vi "Valid Crossings.vi"(8 "Input Valid?":bool, 9 "Value In":fxp<+,32,16> format="%#_21g", 11 "Reference":fxp<+,32,16> format="%#_21g") -> (3 "Value Out":fxp<+,32,16> format="%#_21g")   [LabVIEW 2013]
uses:
  <vilib>/rvi/FXPMathLib/FxpMul/XNode/nifxpmath_Multiplier.xnode
  <vilib>/rvi/FXPMathLib/sim/FxpSim.dll
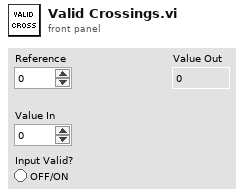
[diagram p1: front panel]
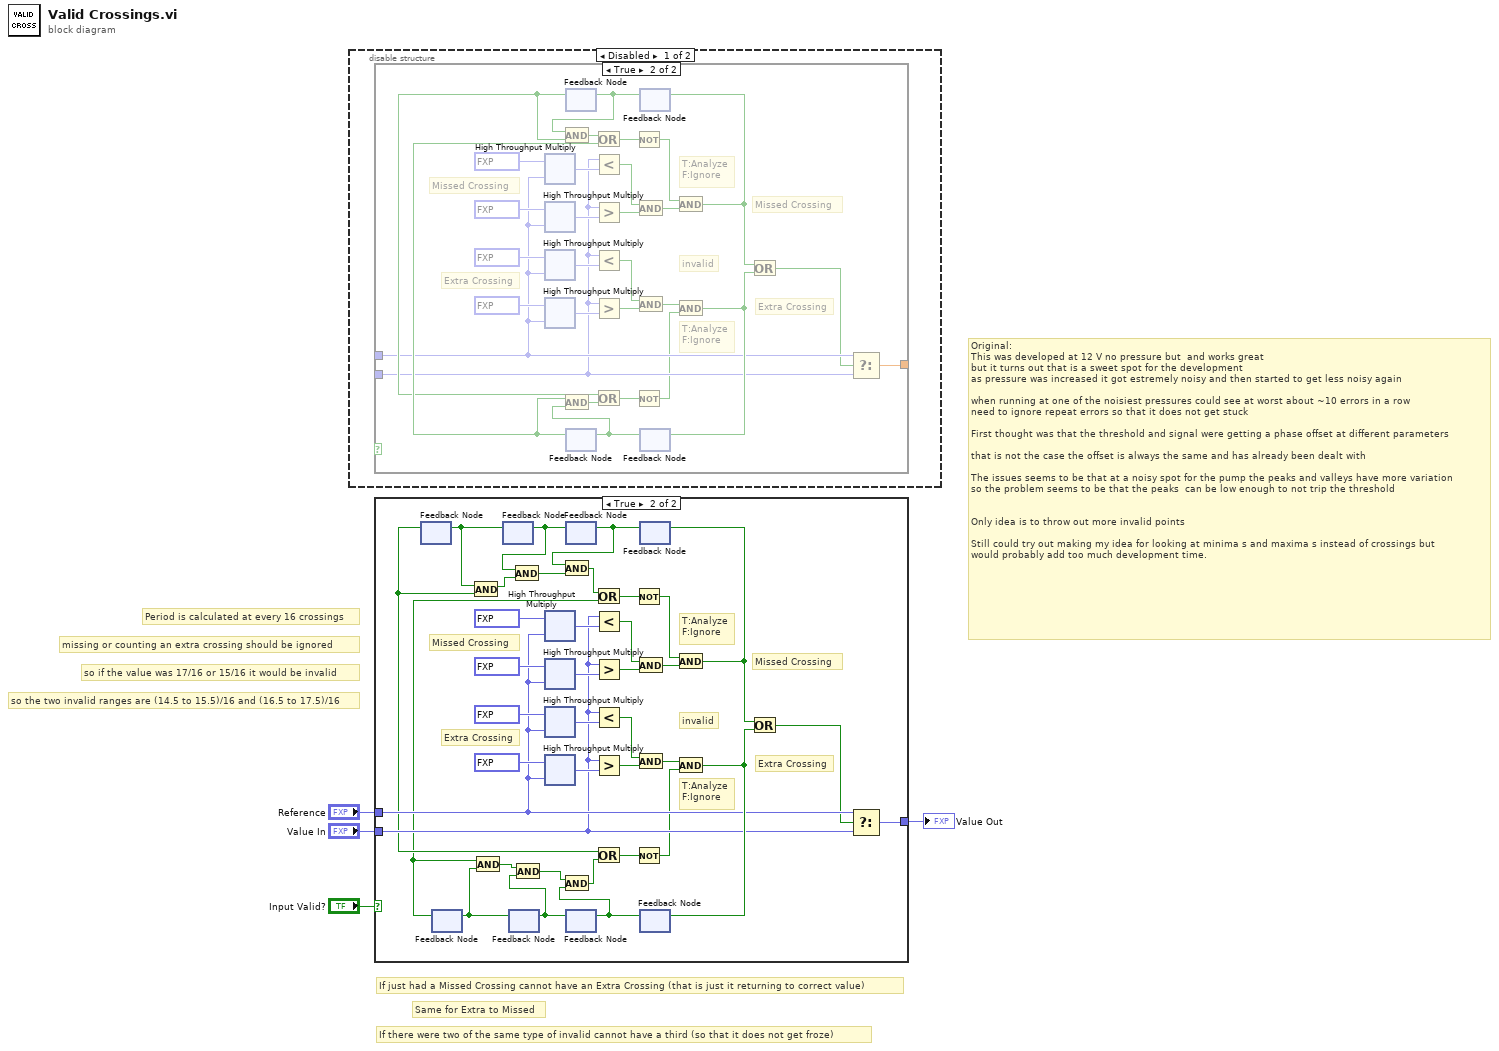
[diagram p0: block diagram]
diagram:
  # "Original:\nThis was developed at 12 V no pressure but  and works great\nbut it turns out that is a sweet spot for the development\nas pressure was increased it got estremely noisy and then started to get less noisy again\n\nwhen running at one of the noisiest pressures could see at worst about ~10 errors in a row\nneed to ignore repeat errors so that it does not get stuck\n\nFirst thought was that the threshold and signal were getting a phase offset at different parameters\n\nthat is not the case the offset is always the same and has already been dealt with\n\nThe issues seems to be that at a noisy spot for the pump the peaks and valleys have more variation\nso the problem seems to be that the peaks  can be low enough to not trip the threshold\n\n\nOnly idea is to throw out more invalid points\n\nStill could try out making my idea for looking at minima s and maxima s instead of crossings but\nwould probably add too much development time."
  # "If there were two of the same type of invalid cannot have a third (so that it does not get froze)"
  # "Same for Extra to Missed"
  # "If just had a Missed Crossing cannot have an Extra Crossing (that is just it returning to correct value)"
  # "so the two invalid ranges are (14.5 to 15.5)/16 and (16.5 to 17.5)/16"
  # "so if the value was 17/16 or 15/16 it would be invalid"
  # "missing or counting an extra crossing should be ignored"
  # "Period is calculated at every 16 crossings"
  n1 = disable-structure shown="Disabled" {
    frame Disabled {
      n2 = case shown="True" {
        selector: _ -> [_ _]
        tunnel: _ -> [w5 w13]
        tunnel: _ -> [_ w11]
        tunnel: [w5 w10] -> _
        frame False {
        }
        frame True {
          # "Missed Crossing"
          # "Extra Crossing"
          # "T:Analyze\nF:Ignore"
          # "T:Analyze\nF:Ignore"
          # "Extra Crossing"
          # "Missed Crossing"
          # "invalid"
          n3 = xnode ("High Throughput Multiply")("x"=fxp<+,6,1> 1.09375, "y"=w13) -> ("x*y"=w31:fxp<+,38,17>)
          n4 = xnode ("High Throughput Multiply")("x"=fxp<+,6,1> 1.03125, "y"=w13) -> ("x*y"=w30:fxp<+,38,17>)
          n5 = xnode ("High Throughput Multiply")("x"=fxp<+,6,1> 0.96875, "y"=w13) -> ("x*y"=w29:fxp<+,38,17>)
          n6 = xnode ("High Throughput Multiply")("x"=fxp<+,6,1> 0.90625, "y"=w13) -> ("x*y"=w28:fxp<+,38,17>)
          n7 = feedback #1() -> (w14:bool)  [unwired: 1 in]
          n8 = feedback #2() -> (w17:bool)  [unwired: 1 in]
          n9 = Less?(x=w11, y=w31) -> (x < y?=w26:bool)
          n10 = Greater?(x=w11, y=w30) -> (0:w27:bool)
          n11 = Less?(x=w11, y=w29) -> (x < y?=w25:bool)
          n12 = Greater?(x=w11, y=w28) -> (0:w24:bool)
          n13 = And(x=w26, y=w27) -> (x .and. y?=w22:bool)
          n14 = And(x=w25, y=w24) -> (x .and. y?=w23:bool)
          n15 = feedback #3() -> (w15:bool)  [unwired: 1 in]
          n16 = And(x=w15, y=w14) -> (x .and. y?=w19:bool)
          n17 = feedback-in #1(w15) -> ()
          n18 = Or(x=w19, y=w17) -> (x .or. y?=w9:bool)
          n19 = Not(x=w9) -> (.not. x?=w6:bool)
          n20 = feedback #4() -> (w16:bool)  [unwired: 1 in]
          n21 = And(x=w17, y=w16) -> (x .and. y?=w18:bool)
          n22 = feedback-in #2(w16) -> ()
          n23 = Or(x=w14, y=w18) -> (x .or. y?=w8:bool)
          n24 = Not(x=w8) -> (.not. x?=w7:bool)
          n25 = And(x=w6, y=w22) -> (x .and. y?=w20:bool)
          n26 = feedback-in #3(w20) -> ()
          n27 = And(x=w23, y=w7) -> (x .and. y?=w21:bool)
          n28 = feedback-in #4(w21) -> ()
          n29 = Or(x=w20, y=w21) -> (x .or. y?=w12:bool)
          n30 = Select(t=w13, s=w12, f=w11) -> (s? t:f=w10:dbl)
        }
      }
    }
    frame Enabled {
    }
  }
  n31 = case shown="True" "Input Valid?" {
    tunnel: "Reference" -> [w36 w54]
    tunnel: "Value In" -> [_ w52]
    tunnel: [w36 w51] -> w2
    frame False {
    }
    frame True {
      # "Missed Crossing"
      # "Extra Crossing"
      # "T:Analyze\nF:Ignore"
      # "T:Analyze\nF:Ignore"
      # "Extra Crossing"
      # "Missed Crossing"
      # "invalid"
      n32 = feedback #5() -> (w46:bool)  [unwired: 1 in]
      n33 = feedback #6() -> (w41:bool)  [unwired: 1 in]
      n34 = feedback #7() -> (w45:bool)  [unwired: 1 in]
      n35 = feedback-in #5(w45) -> ()
      n36 = And(x=w45, y=w46) -> (x .and. y?=w43:bool)
      n37 = feedback #8() -> (w40:bool)  [unwired: 1 in]
      n38 = feedback-in #6(w40) -> ()
      n39 = And(x=w41, y=w40) -> (x .and. y?=w38:bool)
      n40 = xnode ("High Throughput Multiply")("x"=fxp<+,6,1> 1.09375, "y"=w54) -> ("x*y"=w70:fxp<+,38,17>)
      n41 = xnode ("High Throughput Multiply")("x"=fxp<+,6,1> 1.03125, "y"=w54) -> ("x*y"=w69:fxp<+,38,17>)
      n42 = xnode ("High Throughput Multiply")("x"=fxp<+,6,1> 0.96875, "y"=w54) -> ("x*y"=w68:fxp<+,38,17>)
      n43 = xnode ("High Throughput Multiply")("x"=fxp<+,6,1> 0.90625, "y"=w54) -> ("x*y"=w67:fxp<+,38,17>)
      n44 = feedback #9() -> (w44:bool)  [unwired: 1 in]
      n45 = feedback-in #7(w44) -> ()
      n46 = And(x=w44, y=w43) -> (x .and. y?=w42:bool)
      n47 = feedback #10() -> (w39:bool)  [unwired: 1 in]
      n48 = feedback-in #8(w39) -> ()
      n49 = And(x=w38, y=w39) -> (x .and. y?=w37:bool)
      n50 = Less?(x=w52, y=w70) -> (x < y?=w65:bool)
      n51 = Greater?(x=w52, y=w69) -> (0:w66:bool)
      n52 = Less?(x=w52, y=w68) -> (x < y?=w64:bool)
      n53 = Greater?(x=w52, y=w67) -> (0:w63:bool)
      n54 = And(x=w65, y=w66) -> (x .and. y?=w61:bool)
      n55 = And(x=w64, y=w63) -> (x .and. y?=w62:bool)
      n56 = feedback #11() -> (w55:bool)  [unwired: 1 in]
      n57 = And(x=w55, y=w42) -> (x .and. y?=w58:bool)
      n58 = feedback-in #9(w55) -> ()
      n59 = Or(x=w58, y=w41) -> (x .or. y?=w50:bool)
      n60 = Not(x=w50) -> (.not. x?=w47:bool)
      n61 = feedback #12() -> (w56:bool)  [unwired: 1 in]
      n62 = And(x=w37, y=w56) -> (x .and. y?=w57:bool)
      n63 = feedback-in #10(w56) -> ()
      n64 = Or(x=w46, y=w57) -> (x .or. y?=w49:bool)
      n65 = Not(x=w49) -> (.not. x?=w48:bool)
      n66 = And(x=w47, y=w61) -> (x .and. y?=w59:bool)
      n67 = feedback-in #11(w59) -> ()
      n68 = And(x=w62, y=w48) -> (x .and. y?=w60:bool)
      n69 = feedback-in #12(w60) -> ()
      n70 = Or(x=w59, y=w60) -> (x .or. y?=w53:bool)
      n71 = Select(t=w54, s=w53, f=w52) -> (s? t:f=w51:fxp<+,32,16>)
    }
  }
  "Value Out" <- w2
